vi "RT Main.vi"() -> ()   [LabVIEW 2021]
uses:
  <vilib>/Utility/error.llb/Error Cluster From Error Code.vi
  <vilib>/ErrorRing/Error Ring.xnode
  <resource>/objmgr/nicontrollersysapi.rc
panel:
  in  "Abort Button":bool
  in  "Tab Control - Measurement Control":enum32{"Page 2"}(tab)
  in  "Start Measurement Button":bool
  in  "Pause Measurement Button":bool
  in  "Stop Measurement Button":bool
  in  "Tab Control - Configuration":enum32{"Page 2"}(tab)
  in  "Count (uSec)":i32
  in  "Samples per Channel":i32=2000
  out "Timed Out?":bool
  in  "Tab Control - Device Monitoring":enum32{"Page 2"}(tab)
  out "FPGA Temperature [*C]":dbl(slide)=1.0 scale=0.0..85.0
  out "Actual":dbl
  out "Limit":dbl=85.0
  out "PC Host Connected?":bool
  in  "Ring - Menu":u16(ring) items=["Power Analysis", "Harmonics Analysis"]
  # "Measurement Control"
  # "Configuration"
  # "Device Monitoring"
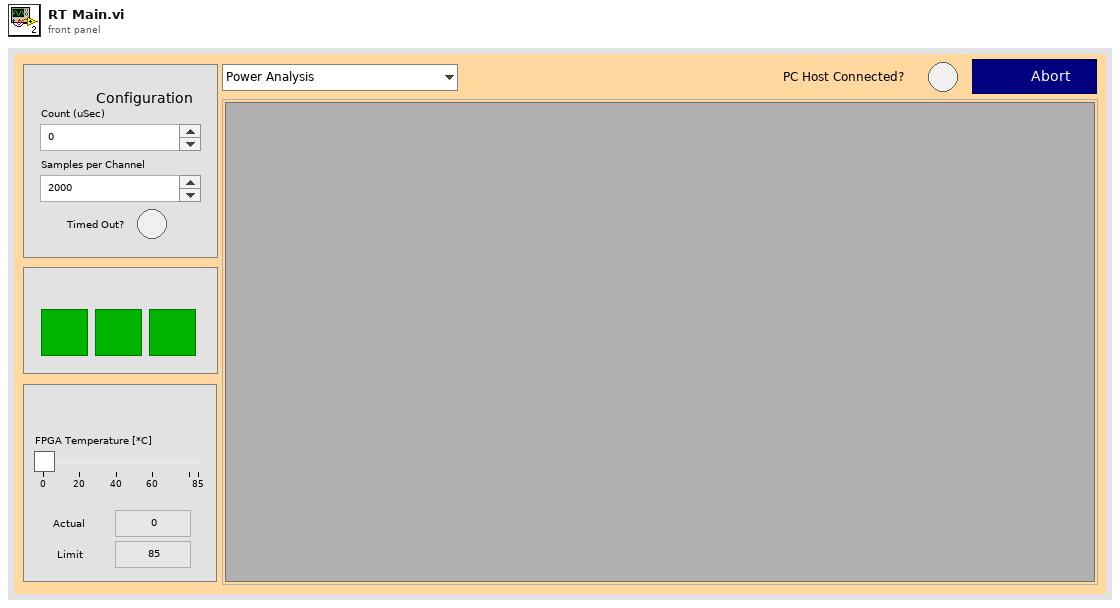
[diagram p1: front panel]
types:
  T1 = typedef "Data - Signals Processing.ctl" = cluster{"SubPanels Ref":refnum<vi>[], "Vi Ref":refnum<vi>}
  T2 = typedef "Data - Error Handler.ctl" = cluster{"message queues":refnum<queue>[], "queue reference - error handler":refnum<queue>, "error":errorcluster}
  T3 = typedef "Data - FPGA Data Acquisition.ctl" = cluster{"Count (uSec)":i32, "Timed Out?":bool, "Samples per Channel":i32}
  T4 = typedef "Data - Command Parser.ctl" = cluster{"PC host connected":bool, "timeout in ms":i32, "reader buffer size":i32, "command":string, "reader endpoint":refnum<k21>}
  T5 = typedef "Data - System Manager.ctl" = cluster{"Stop Avcquisition":bool, "Pause Acquisition":bool, "Start Acquisition":bool, "Type of Acquisition":u16}
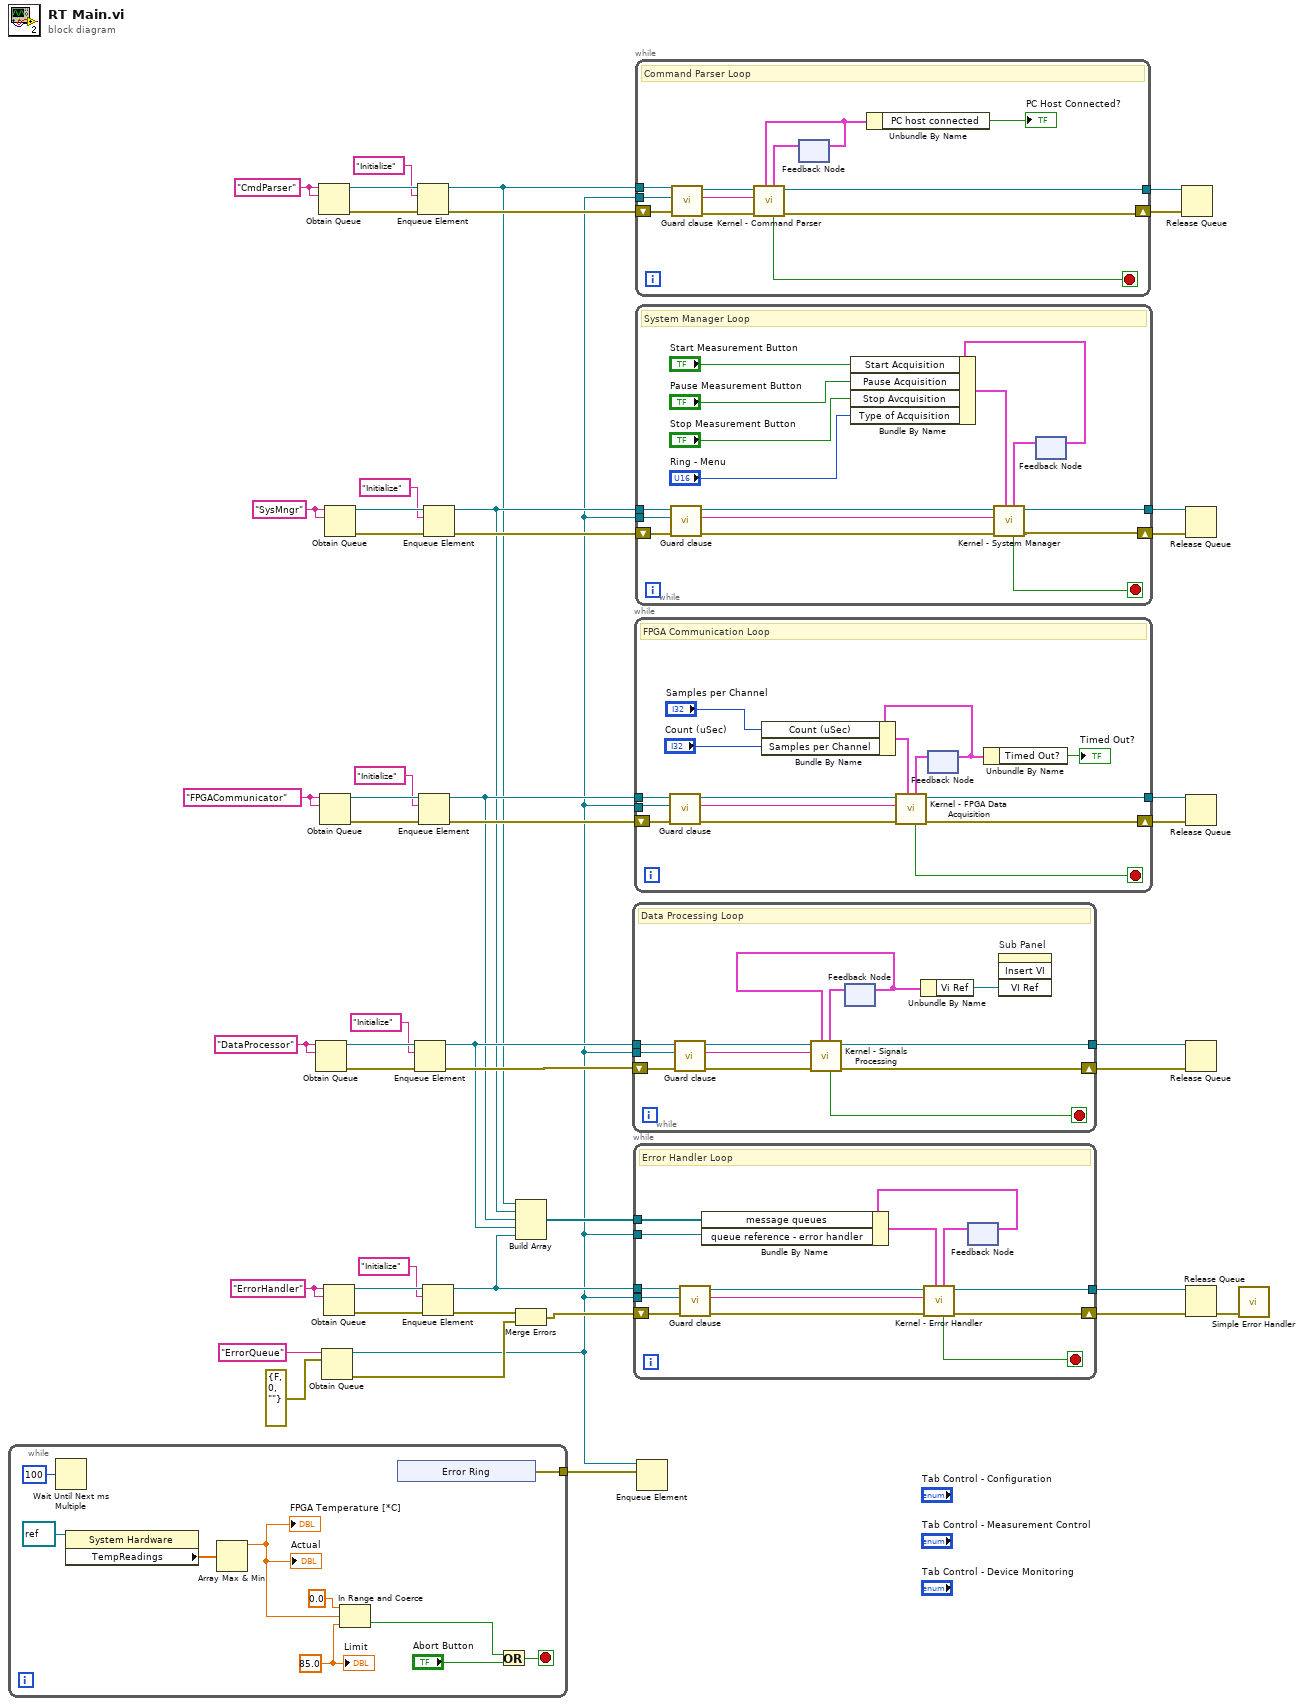
[diagram p0: block diagram]
diagram:
  w14 = "DataProcessor" ("name (unnamed)")
  w21 = "FPGACommunicator" ("name (unnamed)")
  w34 = "ErrorHandler" ("name (unnamed)")
  w41 = "SysMngr" ("name (unnamed)")
  w48 = "CmdParser" ("name (unnamed)")
  n1 = while {
    tunnel: [w57] -> w1
    stop <- w50 stop-if-true
    w53 = 85.0
    n2 = Wait Until Next ms Multiple(millisecond multiple=u32 100) -> ()  [unwired: 1 out]
    n3 = property class="System Hardware"(reference=refnum<k20> refnum ("System Hardware")) -> ("TempReadings"=w54:dbl[])  [unwired: 1 in, 2 out]
    n4 = Array Max & Min(array=w54) -> (max value=w55:dbl)  [unwired: 3 out]
    "FPGA Temperature [*C]" <- w55
    "Actual" <- w55
    n5 = In Range and Coerce(upper limit=0.0, x=w55, lower limit=w53) -> (In Range?=w51:bool)  [unwired: 1 out]
    n6 = xnode "Error Ring"() -> ("error out"=w57:errorcluster)
    n7 = Or(x=w51, y="Abort Button") -> (x .or. y?=w50:bool)
    "Limit" <- w53
  }
  n8 = Obtain Queue(name (unnamed)=w14, element data type=w14) -> (queue out=w12:refnum<queue>, error out=w13:errorcluster)  [unwired: 3 in, 1 out]
  n9 = Obtain Queue(name (unnamed)=w48, element data type=w48) -> (queue out=w46:refnum<queue>, error out=w47:errorcluster)  [unwired: 3 in, 1 out]
  n10 = Obtain Queue(name (unnamed)=w21, element data type=w21) -> (queue out=w19:refnum<queue>, error out=w20:errorcluster)  [unwired: 3 in, 1 out]
  n11 = Obtain Queue(name (unnamed)="ErrorQueue", element data type=errorcluster {"status"=FALSE, "code"=0, "source"=""} ("error out")) -> (queue out=w3:refnum<queue>, error out=w28:errorcluster)  [unwired: 3 in, 1 out]
  n12 = Obtain Queue(name (unnamed)=w34, element data type=w34) -> (queue out=w32:refnum<queue>, error out=w33:errorcluster)  [unwired: 3 in, 1 out]
  n13 = Obtain Queue(name (unnamed)=w41, element data type=w41) -> (queue out=w39:refnum<queue>, error out=w40:errorcluster)  [unwired: 3 in, 1 out]
  n14 = Enqueue Element(queue=w12, element="Initialize", error in (no error)=w13) -> (queue out=w7:refnum<queue>, error out=w10:errorcluster)  [unwired: 1 in, 1 out]
  n15 = Enqueue Element(queue=w46, element="Initialize", error in (no error)=w47) -> (queue out=w4:refnum<queue>, error out=w44:errorcluster)  [unwired: 1 in, 1 out]
  n16 = Enqueue Element(queue=w19, element="Initialize", error in (no error)=w20) -> (queue out=w6:refnum<queue>, error out=w17:errorcluster)  [unwired: 1 in, 1 out]
  n17 = Enqueue Element(queue=w32, element="Initialize", error in (no error)=w33) -> (queue out=w23:refnum<queue>, error out=w30:errorcluster)  [unwired: 1 in, 1 out]
  n18 = Enqueue Element(queue=w39, element="Initialize", error in (no error)=w40) -> (queue out=w5:refnum<queue>, error out=w37:errorcluster)  [unwired: 1 in, 1 out]
  n19 = Build Array(w4, w5, w6, w7, w23) -> (w22:refnum<queue>[])
  n20 = Merge Errors(w30, w28) -> (w27:errorcluster)
  n21 = while {
    tunnel: w7 -> [w75]
    shift-right: [w69] -> w8
    shift-left: w10 -> [w74]
    tunnel: [w68] -> w9
    tunnel: w3 -> [w73]
    stop <- w66 stop-if-true
    # "Data Processing Loop"
    n22 = call "Guard clause.vi"("error in"=w74, "queue - error handler"=w73, "queue - message"=w75) -> ("error out"=w70:errorcluster, "message"=w71:string, "queue out"=w72:refnum<queue>)  [unwired: 6 in]
    n23 = feedback #1() -> (w65:T1)  [unwired: 1 in]
    n24 = call "Kernel - Signals Processing.vi"("data in - Signals Processing"=w65, "error in"=w70, "State"=w71, "message queue"=w72) -> ("error out"=w69:errorcluster, "message queue (out)"=w68:refnum<queue>, "Stop?"=w66:bool, "data out - Signals Processing"=w67:T1)  [unwired: 4 in]
    n25 = feedback-in #1(w67) -> ()
    n26 = Unbundle By Name(w65) -> ("Vi Ref"=w64:refnum<vi>)
    n27 = invoke on="Sub Panel" class="SubPanel" method="Insert VI"("VI Ref"=w64) -> ()  [unwired: 3 in, 4 out]
  }
  n28 = while {
    tunnel: w23 -> [w89]
    shift-right: [w83] -> w25
    shift-left: w27 -> [w88]
    tunnel: w3 -> [w87]
    tunnel: [w84] -> w26
    tunnel: w22 -> [w77]
    tunnel: w3 -> [w76]
    stop <- w82 stop-if-true
    # "Error Handler Loop"
    n29 = call "Guard clause.vi"("error in"=w88, "queue - error handler"=w87, "queue - message"=w89) -> ("error out"=w85:errorcluster, "message"=w81:string, "queue out"=w86:refnum<queue>)  [unwired: 6 in]
    n30 = feedback #2() -> (w79:T2)  [unwired: 1 in]
    n31 = Bundle By Name(cluster=w79, "message queues"=w77, "queue reference - error handler"=w76) -> (w78:T2)
    n32 = call "Kernel - Error Handler.vi"("data in - Error Handler"=w78, "error in"=w85, "State"=w81, "message queue"=w86) -> ("error out"=w83:errorcluster, "message queue (out)"=w84:refnum<queue>, "Stop?"=w82:bool, "data out - Error Handler"=w80:T2)  [unwired: 4 in]
    n33 = feedback-in #2(w80) -> ()
  }
  n34 = while {
    tunnel: w6 -> [w104]
    shift-right: [w97] -> w16
    shift-left: w17 -> [w103]
    tunnel: [w98] -> w15
    tunnel: w3 -> [w102]
    stop <- w92 stop-if-true
    # "FPGA Communication Loop"
    n35 = call "Guard clause.vi"("error in"=w103, "queue - error handler"=w102, "queue - message"=w104) -> ("error out"=w99:errorcluster, "message"=w100:string, "queue out"=w101:refnum<queue>)  [unwired: 6 in]
    n36 = feedback #3() -> (w94:T3)  [unwired: 1 in]
    n37 = Bundle By Name(cluster=w94, "Count (uSec)"="Samples per Channel", "Samples per Channel"="Count (uSec)") -> (w93:T3)
    n38 = call "Kernel - FPGA Data Acquisition.vi"("Data in - FPGA Data Acquisition"=w93, "error in"=w99, "State"=w100, "message queue"=w101) -> ("error out"=w97:errorcluster, "message queue (out)"=w98:refnum<queue>, "Stop?"=w92:bool, "Data out - FPGA Data Acquisition"=w96:T3)  [unwired: 4 in]
    n39 = feedback-in #3(w96) -> ()
    n40 = Unbundle By Name(w94) -> ("Timed Out?"=→"Timed Out?":bool)
  }
  n41 = while {
    tunnel: w4 -> [w116]
    shift-right: [w111] -> w43
    shift-left: w44 -> [w115]
    tunnel: [w110] -> w42
    tunnel: w3 -> [w114]
    stop <- w109 stop-if-true
    # "Command Parser Loop"
    n42 = call "Guard clause.vi"("error in"=w115, "queue - error handler"=w114, "queue - message"=w116) -> ("error out"=w112:errorcluster, "message"=w106:string, "queue out"=w113:refnum<queue>)  [unwired: 6 in]
    n43 = feedback #4() -> (w107:T4)  [unwired: 1 in]
    n44 = call "Kernel - Command Parser.vi"("data in - Command Parser"=w107, "error in"=w112, "state"=w106, "message queue"=w113) -> ("error out"=w111:errorcluster, "message queue (out)"=w110:refnum<queue>, "stop?"=w109:bool, "data out - Command Parser"=w108:T4)  [unwired: 4 in]
    n45 = feedback-in #4(w108) -> ()
    n46 = Unbundle By Name(w107) -> ("PC host connected"=→"PC Host Connected?":bool)
  }
  n47 = while {
    tunnel: w5 -> [w132]
    shift-right: [w128] -> w36
    shift-left: w37 -> [w131]
    tunnel: [w126] -> w35
    tunnel: w3 -> [w130]
    stop <- w124 stop-if-true
    # "System Manager Loop"
    n48 = call "Guard clause.vi"("error in"=w131, "queue - error handler"=w130, "queue - message"=w132) -> ("error out"=w129:errorcluster, "message"=w125:string, "queue out"=w127:refnum<queue>)  [unwired: 6 in]
    n49 = feedback #5() -> (w122:T5)  [unwired: 1 in]
    n50 = Bundle By Name(cluster=w122, "Start Acquisition"="Start Measurement Button", "Pause Acquisition"="Pause Measurement Button", "Stop Avcquisition"="Stop Measurement Button", "Type of Acquisition"="Ring - Menu") -> (w121:T5)
    n51 = call "Kernel - System Manager.vi"("Data in - System Manager"=w121, "error in"=w129, "State"=w125, "message queue"=w127) -> ("error out"=w128:errorcluster, "message queue (out)"=w126:refnum<queue>, "Stop?"=w124:bool, "Data out - System Manager"=w123:T5)  [unwired: 4 in]
    n52 = feedback-in #5(w123) -> ()
  }
  n53 = Enqueue Element(queue=w3, element=w1) -> ()  [unwired: 2 in, 3 out]
  n54 = Release Queue(queue=w42, error in (no error)=w43) -> ()  [unwired: 1 in, 3 out]
  n55 = Release Queue(queue=w35, error in (no error)=w36) -> ()  [unwired: 1 in, 3 out]
  n56 = Release Queue(queue=w15, error in (no error)=w16) -> ()  [unwired: 1 in, 3 out]
  n57 = Release Queue(queue=w9, error in (no error)=w8) -> ()  [unwired: 1 in, 3 out]
  n58 = Release Queue(queue=w26, error in (no error)=w25) -> (error out=w24:errorcluster)  [unwired: 1 in, 2 out]
  n59 = call <vilib>:"Simple Error Handler.vi"("error in (no error)"=w24) -> ()  [unwired: 4 in, 5 out]
